vi "(TestVI)DW7912 Memory Converting.vi"() -> ()   [LabVIEW 2020]
panel:
  out "최소 인덱스 addr":i32
  out "최소값 addr":u16
  out "최대 인덱스 addr":i32
  out "최대값 addr":u16
  out "최소 인덱스 size":i32
  out "최소값 size":u16
  out "최대 인덱스 size":i32
  out "최대값 size":u16
  in  "정지":bool
  in  "인덱스 (행)":i32
  out "웨이브폼 그래프":i8[](graph)
  out "클러스터":T1 {"VD Clamp" format="0x%02x    %d"; "Wave Size" format="0x%04x    %d"; "Wait" format="0x%02x    %d"; "Start Address" format="0x%04x    %d"}
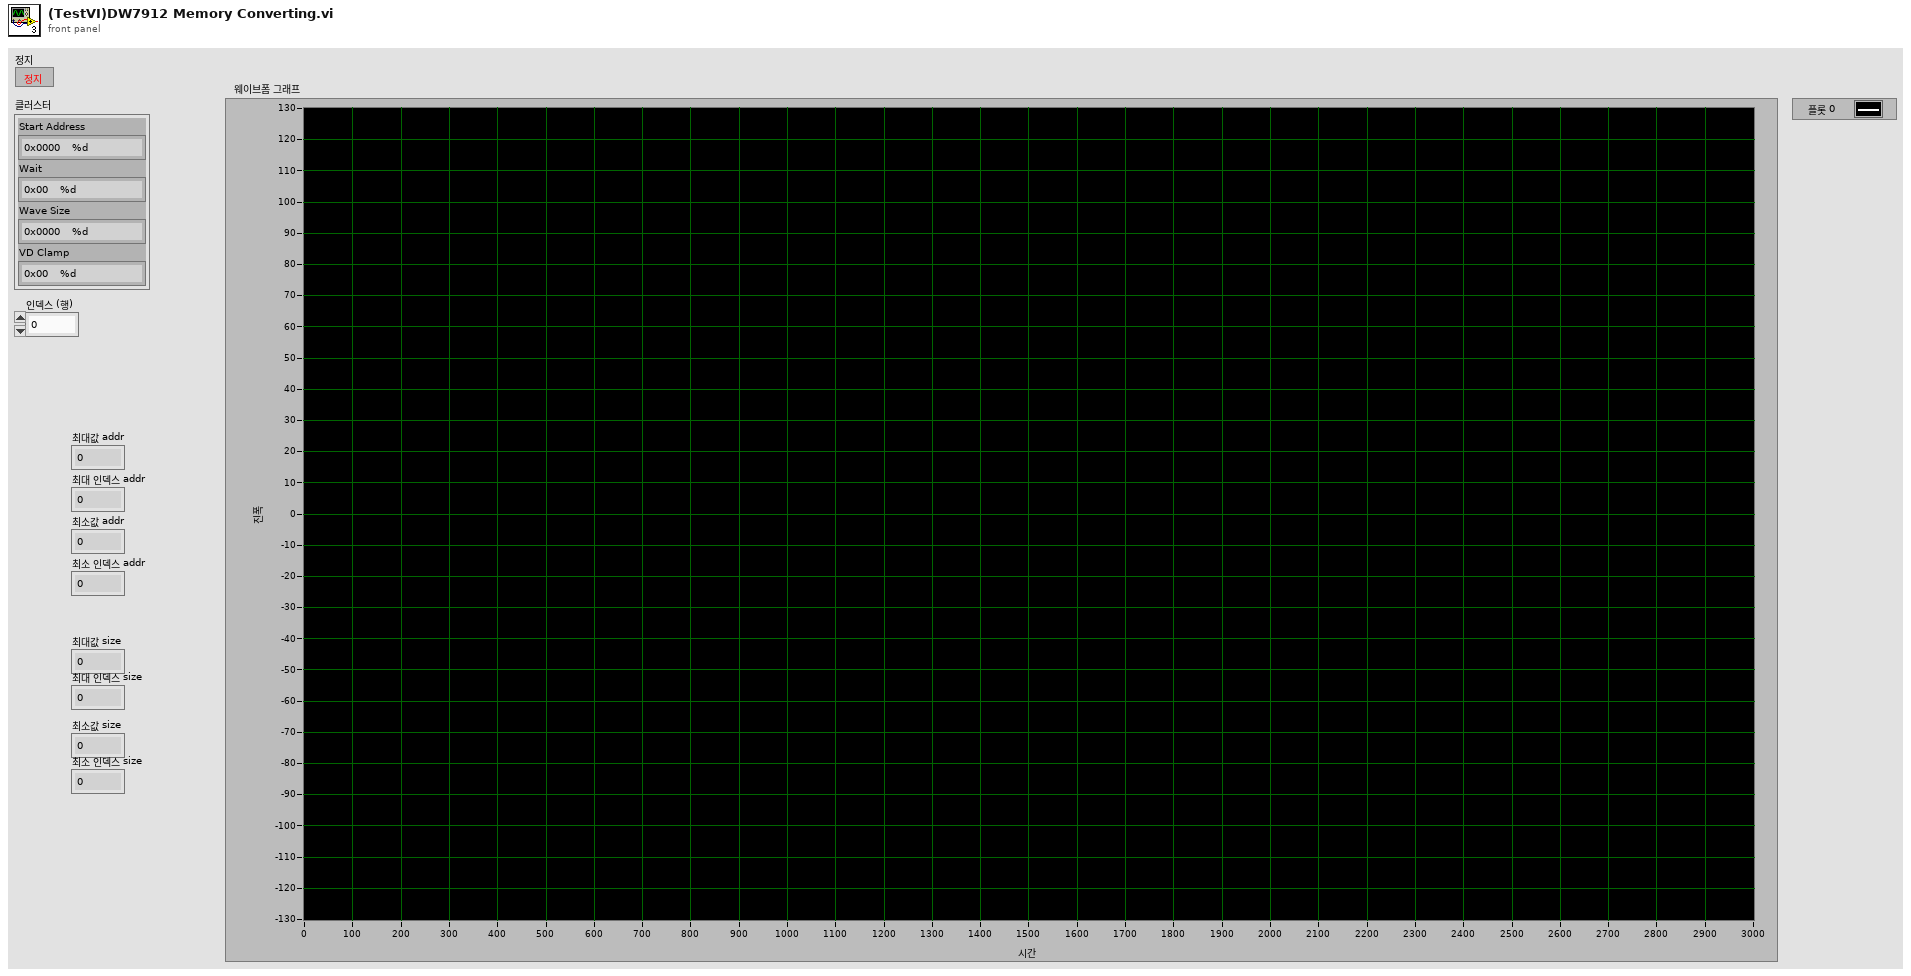
[diagram p1: front panel]
types:
  T1 = cluster{"Start Address":u16, "Wait":u8, "Wave Size":u16, "VD Clamp":u8}
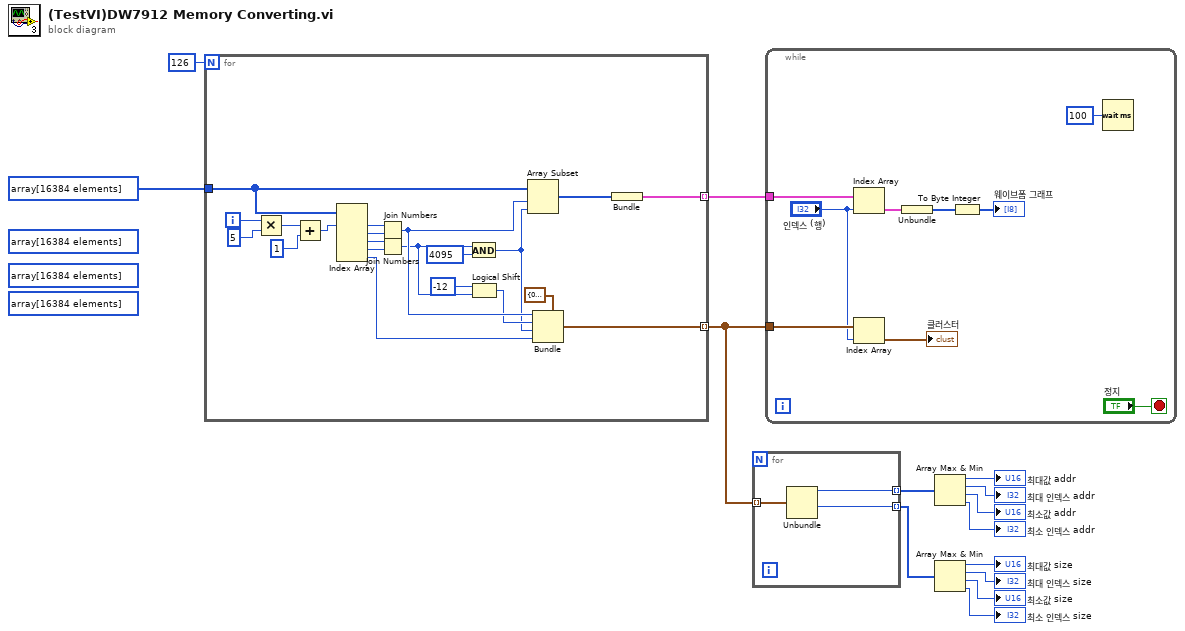
[diagram p0: block diagram]
diagram:
  (unwired) u8[] array[16384 elements] ("Read Data")
  (unwired) u8[] array[16384 elements] ("Read Data")
  (unwired) u8[] array[16384 elements] ("Read Data")
  n1 = for {
    N: 126 -> [_]
    tunnel: u8[] array[16384 elements] ("Read Data") -> [w26]
    tunnel: [w17] -> w12 mode=indexing
    tunnel: [w15] -> w13 mode=indexing
    i -> [w35]
    n2 = Multiply(x=w35, y=5) -> (x*y=w33:i32)
    n3 = Add(x=w33, y=1) -> (x+y=w28:i32)
    n4 = Index Array(array=w26, index #1=w28) -> (element #1=w32:u8, element #2=w31:u8, element #3=w30:u8, element #4=w29:u8, element #5=w18:u8)  [unwired: 4 in]
    n5 = Join Numbers(hi=w32, lo=w31) -> ((hi.lo)=w24:u16)
    n6 = Join Numbers(hi=w30, lo=w29) -> ((hi.lo)=w22:u16)
    n7 = And(x=w22, y=u16 4095) -> (x .and. y?=w19:u16)
    n8 = Logical Shift(y=i16 -12, x=w22) -> (x << y=w20:u16)
    n9 = Array Subset(array=w26, index=w24, length=w19) -> (w16:u8[])
    n10 = Bundle(cluster=T1 {"Start Address"=0, "Wait"=0, "Wave Size"=0, "VD Clamp"=0} ("클러스터"), "Start Address"=w24, "Wait"=w20, "Wave Size"=w19, "VD Clamp"=w18) -> (w17:T1)
    n11 = Bundle(w16) -> (w15:cluster{u8[]})  [unwired: 1 in]
  }
  n12 = for {
    tunnel: w12 -> [w38] mode=indexing
    tunnel: [w37] -> w11 mode=indexing
    tunnel: [w36] -> w10 mode=indexing
    n13 = Unbundle(w38) -> ("Start Address"=w37:u16, "Wave Size"=w36:u16)  [unwired: 2 out]
  }
  n14 = while {
    tunnel: w13 -> [w47]
    tunnel: w12 -> [w46]
    stop <- "정지" stop-if-true
    n15 = Index Array(array=w47, index="인덱스 (행)") -> (element=w44:cluster{u8[]})
    n16 = Index Array(array=w46, index="인덱스 (행)") -> (element=→"클러스터":T1)
    n17 = Unbundle(w44) -> (w40:u8[])
    n18 = To Byte Integer(number=w40) -> (8bit integer=→"웨이브폼 그래프":i8[])
    n19 = Wait (ms)(milliseconds to wait=u32 100 ("대기 시간 (ms)")) -> ()  [unwired: 1 out]
  }
  n20 = Array Max & Min(array=w11) -> (max value=→"최대값 addr":u16, max index (indices)=→"최대 인덱스 addr":i32, min value=→"최소값 addr":u16, min index (indices)=→"최소 인덱스 addr":i32)
  n21 = Array Max & Min(array=w10) -> (max value=→"최대값 size":u16, max index (indices)=→"최대 인덱스 size":i32, min value=→"최소값 size":u16, min index (indices)=→"최소 인덱스 size":i32)
